vi "Get Steps.vi"(8 "error in (no error)":errorcluster, 11 "Sequence in":refnum<class "Sequence.lvclass">) -> (0 "error out":errorcluster, 2 "Steps":refnum<class "Step.lvclass">[](array[class]), 3 "Sequence out":refnum<class "Sequence.lvclass">)   [LabVIEW 2020, in "Tester.lvlib" / "Sequence.lvclass"]
uses:
  Sequence.lvclass
  Step/Step.lvclass
  Sequence.lvclass/Sequence.ctl
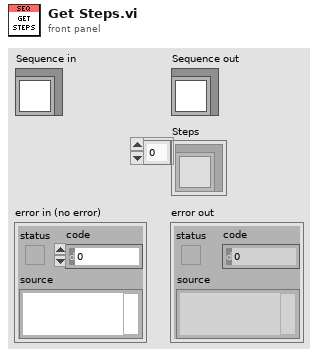
[diagram p1: front panel]
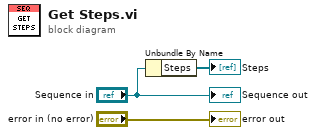
[diagram p0: block diagram]
diagram:
  n1 = Unbundle By Name("Sequence in") -> ("Steps"=→"Steps":refnum<class "Step.lvclass">[])
  "error out" <- "error in (no error)"
  "Sequence out" <- "Sequence in"
